vi "Create Trigger Channel.vi"(8 "error in (no error)":errorcluster, 10 "Channel Parameters":T1, 11 "Message Channels Section in":T3 format="%.0x") -> (0 "error out":errorcluster, 3 "Message Channels Section out":T3 format="%.0x")   [LabVIEW 2018, in "Instrument Addon Scripting API.lvlib"]
uses:
  Instrument Addon Scripting API.lvlib
  <vilib>/NI Veristand/Custom Device API/Custom Device Item Ref.ctl
  <vilib>/NI Veristand/Custom Device API/Custom Device Channel.ctl
  <vilib>/NI Veristand/Custom Device API/Custom Device Channel Type.ctl
  Addon/Addon Shared/SubVIs/Constants.vi
  Addon/Addon Shared/Instrument Addon Shared.lvlib
  <vilib>/NI Veristand/Custom Device API/Custom Device API.lvlib
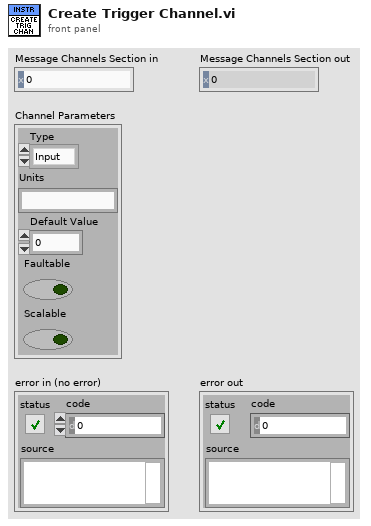
[diagram p1: front panel]
types:
  T1 = typedef "Custom Device API.lvlib/Custom Device Channel.ctl" = cluster{"Type":T2, "Units":string, "Default Value":dbl, "Faultable":bool, "Scalable":bool}
  T2 = typedef "Custom Device API.lvlib/Custom Device Channel Type.ctl" = enum16{"Input", "Output"}
  T3 = typedef "Custom Device API.lvlib/Custom Device Item Ref.ctl" = u64
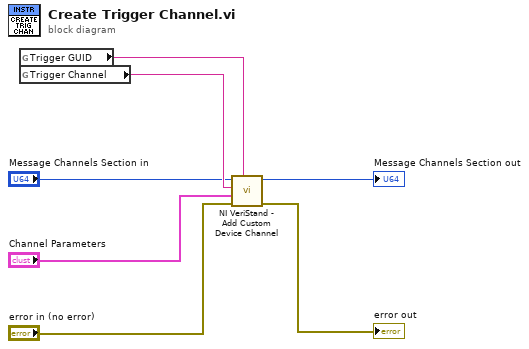
[diagram p0: block diagram]
diagram:
  n1 = global read "Constants.vi" "Trigger GUID"() -> (w4:string)
  n2 = global read "Constants.vi" "Trigger Channel"() -> (w5:string)
  n3 = call <vilib>:"NI VeriStand - Add Custom Device Channel.vi"("GUID (Default Channel)"=w4, "error in (no error)"="error in (no error)", "Channel"="Channel Parameters", "Channel Name"=w5, "Parent Ref in"="Message Channels Section in") -> ("error out"=→"error out":errorcluster, "Parent Ref out"=→"Message Channels Section out":T3)  [unwired: 3 in, 2 out]
